vi "PicoScopeospaAWG.vi"(0 "Handle In":i16=16384, 1 "General AWG Settings":T4={"Peak-to-Peak Voltage"=2.0, "Offset Voltage"=0.0, "Wave Type"=17, "Sweep Type"=0, "Cycles"=10, "Trigger Type"=0, "Trigger Source"=4, "sigGenEnabled"=TRUE, "Trigger Enabled"=FALSE, "autoTriggerPicoSeconds"=0} {"Trigger Source" items=["None"=0, "Scope Trigger"=1, "Software Trigger"=4, "Trigger Raw"=5]; "Trigger Type" items=["Rising", "Falling", "Gate High", "Gate Low"]; "Sweep Type" items=["Up", "Down", "Up-Down", "Down-Up"]; "Wave Type" items=["Sine"=17, "Square"=18, "Triangle"=19, "Ramp Up"=20, "Ramp Down"=21, "Sinc"=22, "Gaussian"=23, "Half Sine"=24, "DC"=1024, "PWM"=4096, "White Noise"=8193, "PRBS"=8194, "Arbitrary"=268435456]; "Offset Voltage" format="%#_6p"; "Peak-to-Peak Voltage" format="%#_6p"}, 2 "Standard Waveform Settings":T3={"(Start) Frequency"=1000.0, "Stop Frequency"=5000.0, "Increment"=1.0, "Dwell Time (seconds)"=0.001, "Sweep Enabled"=FALSE} {"Dwell Time (seconds)" format="%#_6p"; "Stop Frequency" min=0.03 max=1000000.0 format="%#_6p"; "(Start) Frequency" min=0.03 max=1000000.0 format="%#_6p"}, 3 "Arbitrary Waveform Settings":T2 {"Index Mode" items=["Single", "Dual", "Quad"]}, 11 "error in":errorcluster, 12 "Duty Cycle":T1={"Use Duty Cycle"=FALSE, "dutyCyclePercent"=20.0}) -> (4 "Handle Out":i16=16384, 13 "Trigger Source Out":u32=4, 14 "Arbitrary\nWaveform Graph":i16[](graph), 15 "error out":errorcluster)   [LabVIEW 2010]
doc: "This VI can be used to control the arbitrary waveform generator. Standard waveforms can be selected or arbitrary waveform can be selected under 'Wave Type'. There are three settings clusters: general settings that apply to both arbitrary and standard waveforms, settings that apply only to standard waveforms and settings that apply only to arbitrary waveforms. It is not necessary to connect all of these clusters if only using arbitrary waveforms or only using standard waveforms are required.\n\nWhen selecting arbitrary waveform, it is necessary to specify a text file containing the wave form. This text file should have a single value on each line in the range -1 to 1. For further information on the settings, see descriptions of ps3000aSetSigGenBuiltIn and ps3000aSetSigGenArbitrary."
uses:
  psospa.dll
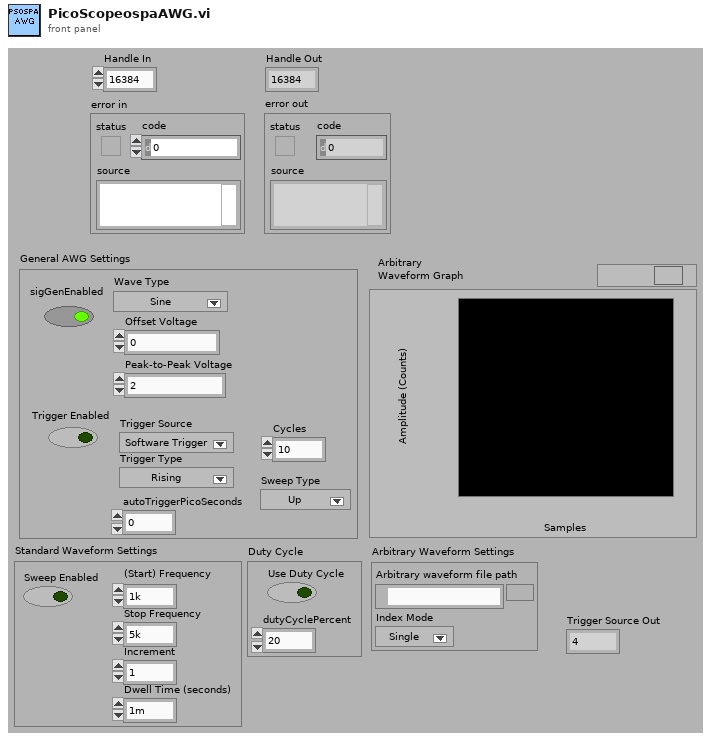
[diagram p1: front panel]
types:
  T1 = cluster{"Use Duty Cycle":bool, "dutyCyclePercent":dbl}
  T2 = cluster{"Arbirary waveform file path":path, "Index Mode":u32}
  T3 = cluster{"(Start) Frequency":dbl, "Stop Frequency":dbl, "Increment":dbl, "Dwell Time (seconds)":dbl, "Sweep Enabled":bool}
  T4 = cluster{"Peak-to-Peak Voltage":dbl, "Offset Voltage":dbl, "Wave Type":u32, "Sweep Type":u32, "Cycles":u64, "Trigger Type":u32, "Trigger Source":u32, "sigGenEnabled":bool, "Trigger Enabled":bool, "autoTriggerPicoSeconds":u64}
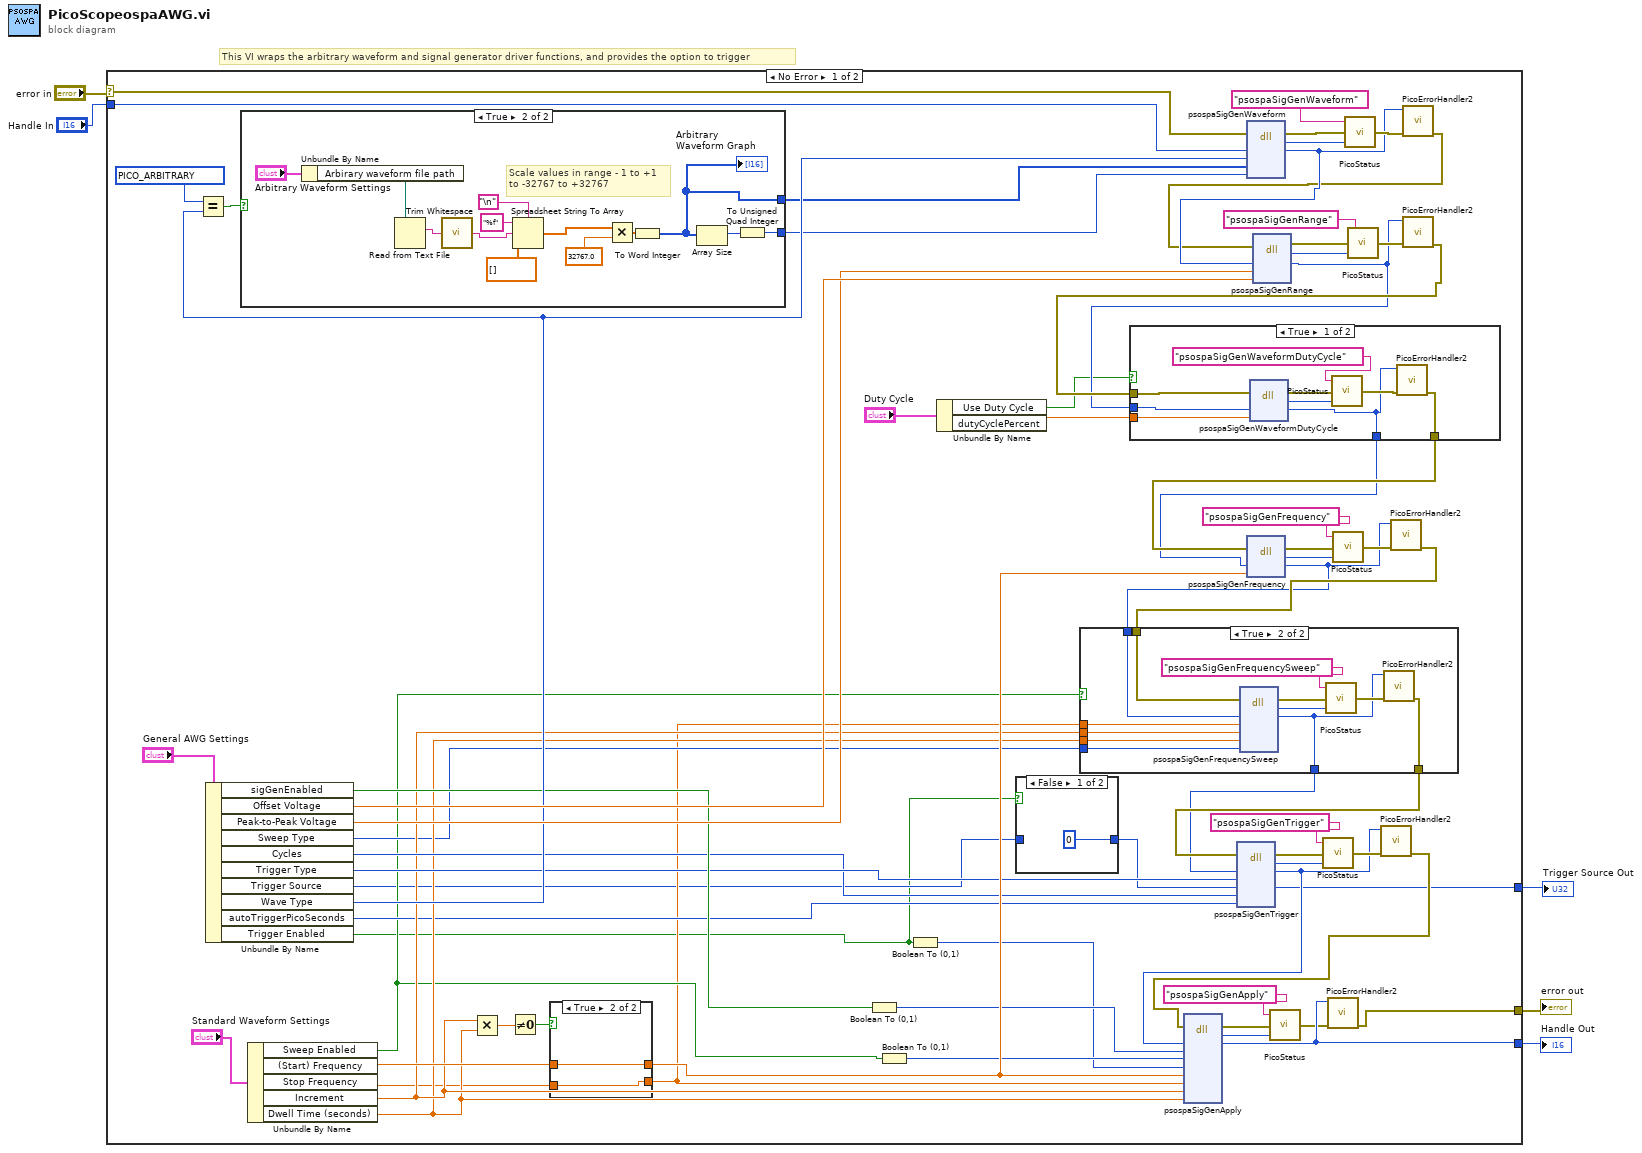
[diagram p0: block diagram]
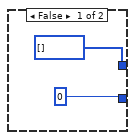
[diagram p4: hidden frame]
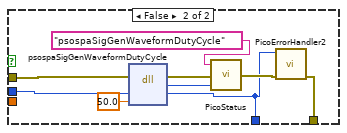
[diagram p5: hidden frame]
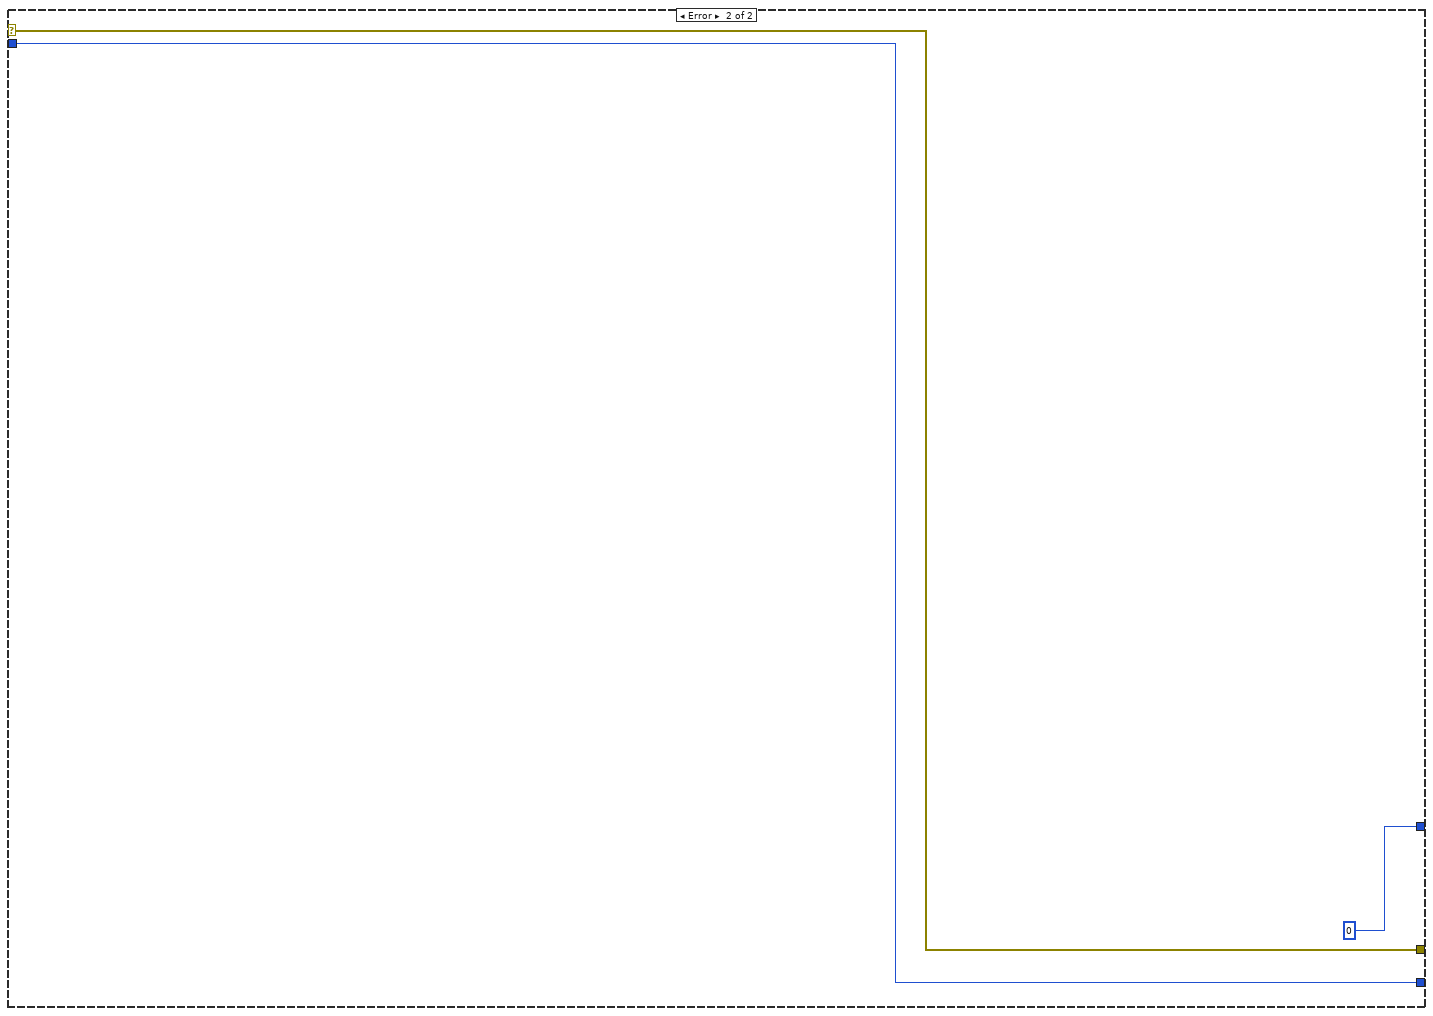
[diagram p7: hidden frame]
diagram:
  # "This VI wraps the arbitrary waveform and signal generator driver functions, and provides the option to trigger"
  n1 = case shown="No Error" "error in" {
    selector: "error in" -> [w69 w129]
    tunnel: [w63 w128] -> w5
    tunnel: "Handle In" -> [w74 w128]
    tunnel: [w62 w129] -> w3
    tunnel: [w9 0] -> w1
    frame No Error {
      w61 = u32 268435456 items=["PICO_ARBITRARY"=268435456]
      n2 = Unbundle By Name("General AWG Settings") -> ("sigGenEnabled"=w32:bool, "Offset Voltage"=w72:dbl, "Peak-to-Peak Voltage"=w71:dbl, "Sweep Type"=w13:u32, "Cycles"=w21:u64, "Trigger Type"=w22:u32, "Trigger Source"=w7:u32, "Wave Type"=w70:u32, "autoTriggerPicoSeconds"=w12:u64, "Trigger Enabled"=w6:bool)
      n3 = Equal?(x=w61, y=w70) -> (x = y?=w33:bool)
      n4 = case shown="True" w33 {
        tunnel: [i16[] [] ("buffer") w94] -> w42
        tunnel: [u64 0 ("bufferLenght") w93] -> w34
        frame False {
        }
        frame True {
          # "Scale values in range - 1 to +1 \nto -32767 to +32767"
          n5 = Unbundle By Name("Arbitrary Waveform Settings") -> ("Arbirary waveform file path"=w99:path)
          n6 = Read from Text File(file (use dialog)=w99) -> (text=w97:string)  [unwired: 3 in, 3 out]
          n7 = call <vilib>:"Trim Whitespace.vi"("string"=w97) -> ("trimmed string"=w96:string)  [unwired: 1 in]
          n8 = Spreadsheet String To Array(delimiter (Tab)="\n", format string="%f", spreadsheet string=w96, array type (2D Dbl)=dbl[] []) -> (array=w101:dbl[])
          n9 = Multiply(x=w101, y=32767.0 ("deltaPhaseIncrement")) -> (x*y=w98:dbl[])
          n10 = To Word Integer(number=w98) -> (16bit integer=w94:i16[])
          "Arbitrary\nWaveform Graph" <- w94
          n11 = Array Size(array=w94) -> (size(s)=w95:i32)
          n12 = To Unsigned Quad Integer(1:w95) -> (0:w93:u64)
        }
      }
      n13 = Unbundle By Name("Standard Waveform Settings") -> ("Sweep Enabled"=w11:bool, "(Start) Frequency"=w67:dbl, "Stop Frequency"=w18:dbl, "Increment"=w20:dbl, "Dwell Time (seconds)"=w19:dbl)
      n14 = Multiply(x=w20, y=w19) -> (x*y=w66:dbl)
      n15 = Not Equal To 0?(x=w66) -> (x != 0?=w65:bool)
      n16 = case shown="True" w65 {
        tunnel: [w124 w126] -> w10
        tunnel: w18 -> [_ w126]
        tunnel: w67 -> [w124 w125]
        tunnel: [w124 w125] -> w64
        frame False {
        }
        frame True {
        }
      }
      n17 = Boolean To (0,1)(Boolean=w32) -> (0, 1=w37:i16)
      n18 = Boolean To (0,1)(Boolean=w11) -> (0, 1=w36:i16)
      n19 = Boolean To (0,1)(Boolean=w6) -> (0, 1=w35:i16)
      n20 = Unbundle By Name("Duty Cycle") -> ("Use Duty Cycle"=w30:bool, "dutyCyclePercent"=w29:dbl)
      n21 = case shown="False" w6 {
        tunnel: [u32 0 ("Trigger Source") w76] -> w8
        tunnel: w7 -> [_ w76]
        frame False {
        }
        frame True {
        }
      }
      n22 = dll-call lib="psospa.dll" fn="psospaSigGenWaveform" ("ps3000.dll:_ps3000_open_unit@0")(error in=w69, "handle"=w74, "waveType"=w70, "buffer"=w42, "bufferLenght"=w34) -> (error out=w58:errorcluster, "PICO_STATUS"=w50:u32, "handle"=w55:i16)  [unwired: 5 in, 1 out]
      n23 = call "PicoStatus.vi"("PICO STATUS"=w50, "error in"=w58, "source"="psospaSigGenWaveform") -> ("error out"=w57:errorcluster)
      n24 = call "PicoErrorHandler2.vi"("error in (no error)"=w57, "handle In"=w55) -> ("error out"=w54:errorcluster)  [unwired: 9 in]
      n25 = dll-call lib="psospa.dll" fn="psospaSigGenRange" ("ps3000.dll:_ps3000_open_unit@0")(error in=w54, "handle"=w55, "peakToPeakVolts"=w71, "offsetVolts"=w72) -> (error out=w53:errorcluster, "PICO_STATUS"=w51:u32, "handle"=w48:i16)  [unwired: 4 in, 1 out]
      n26 = call "PicoStatus.vi"("PICO STATUS"=w51, "error in"=w53, "source"="psospaSigGenRange") -> ("error out"=w52:errorcluster)
      n27 = call "PicoErrorHandler2.vi"("error in (no error)"=w52, "handle In"=w48) -> ("error out"=w49:errorcluster)  [unwired: 9 in]
      n28 = case shown="True" w30 {
        tunnel: w49 -> [w111 w120]
        tunnel: w48 -> [w110 w119]
        tunnel: [w109 w118] -> w46
        tunnel: [w108 w117] -> w45
        tunnel: w29 -> [w106 _]
        frame True {
          n29 = dll-call lib="psospa.dll" fn="psospaSigGenWaveformDutyCycle" ("ps3000.dll:_ps3000_open_unit@0")(error in=w111, "handle"=w110, "dutyCyclePercent"=w106) -> (error out=w114:errorcluster, "PICO_STATUS"=w113:u32, "handle"=w108:i16)  [unwired: 3 in, 1 out]
          n30 = call "PicoStatus.vi"("PICO STATUS"=w113, "error in"=w114, "source"="psospaSigGenWaveformDutyCycle") -> ("error out"=w112:errorcluster)
          n31 = call "PicoErrorHandler2.vi"("error in (no error)"=w112, "handle In"=w108) -> ("error out"=w109:errorcluster)  [unwired: 9 in]
        }
        frame False {
          n32 = dll-call lib="psospa.dll" fn="psospaSigGenWaveformDutyCycle" ("ps3000.dll:_ps3000_open_unit@0")(error in=w120, "handle"=w119, "dutyCyclePercent"=50.0) -> (error out=w123:errorcluster, "PICO_STATUS"=w122:u32, "handle"=w117:i16)  [unwired: 3 in, 1 out]
          n33 = call "PicoStatus.vi"("PICO STATUS"=w122, "error in"=w123, "source"="psospaSigGenWaveformDutyCycle") -> ("error out"=w121:errorcluster)
          n34 = call "PicoErrorHandler2.vi"("error in (no error)"=w121, "handle In"=w117) -> ("error out"=w118:errorcluster)  [unwired: 9 in]
        }
      }
      n35 = dll-call lib="psospa.dll" fn="psospaSigGenFrequency" ("ps3000.dll:_ps3000_open_unit@0")(error in=w46, "handle"=w45, "frequencyHz"=w64) -> (error out=w60:errorcluster, "PICO_STATUS"=w59:u32, "handle"=w16:i16)  [unwired: 3 in, 1 out]
      n36 = call "PicoStatus.vi"("PICO STATUS"=w59, "error in"=w60, "source"="psospaSigGenFrequency") -> ("error out"=w47:errorcluster)
      n37 = call "PicoErrorHandler2.vi"("error in (no error)"=w47, "handle In"=w16) -> ("error out"=w17:errorcluster)  [unwired: 9 in]
      n38 = case shown="True" w11 {
        tunnel: w20 -> [_ w86]
        tunnel: w19 -> [_ w85]
        tunnel: w10 -> [_ w84]
        tunnel: w17 -> [w77 w83]
        tunnel: w16 -> [w78 w82]
        tunnel: [w77 w81] -> w15
        tunnel: [w78 w80] -> w14
        tunnel: w13 -> [_ w79]
        frame False {
        }
        frame True {
          n39 = dll-call lib="psospa.dll" fn="psospaSigGenFrequencySweep" ("ps3000.dll:_ps3000_open_unit@0")(error in=w83, "handle"=w82, "stopFrequencyHz"=w84, "frequencyIncrement"=w86, "dwellTimeSeconds"=w85, "sweepType"=w79) -> (error out=w90:errorcluster, "PICO_STATUS"=w89:u32, "handle"=w80:i16)  [unwired: 6 in, 1 out]
          n40 = call "PicoStatus.vi"("PICO STATUS"=w89, "error in"=w90, "source"="psospaSigGenFrequencySweep") -> ("error out"=w88:errorcluster)
          n41 = call "PicoErrorHandler2.vi"("error in (no error)"=w88, "handle In"=w80) -> ("error out"=w81:errorcluster)  [unwired: 9 in]
        }
      }
      n42 = dll-call lib="psospa.dll" fn="psospaSigGenTrigger" ("ps3000.dll:_ps3000_open_unit@0")(error in=w15, "handle"=w14, "triggerType"=w22, "triggerSource"=w8, "cycles"=w21, "autoTriggerPicoSeconds"=w12) -> (error out=w28:errorcluster, "PICO_STATUS"=w27:u32, "handle"=w23:i16, "triggerSource"=w9:u32)  [unwired: 5 in, 1 out]
      n43 = call "PicoStatus.vi"("PICO STATUS"=w27, "error in"=w28, "source"="psospaSigGenTrigger") -> ("error out"=w26:errorcluster)
      n44 = call "PicoErrorHandler2.vi"("error in (no error)"=w26, "handle In"=w23) -> ("error out"=w24:errorcluster)  [unwired: 9 in]
      n45 = dll-call lib="psospa.dll" fn="psospaSigGenApply" ("ps3000.dll:_ps3000_open_unit@0")(error in=w24, "handle"=w23, "sigGenEnabled"=w37, "sweepEnabled"=w36, "triggerEnabled"=w35, "frequency"=w64, "stopFrequency"=w10, "frequencyIncrement"=w20, "dwellTime"=w19) -> (error out=w41:errorcluster, "PICO_STATUS"=w40:u32, "handle"=w63:i16)  [unwired: 9 in, 1 out]
      n46 = call "PicoStatus.vi"("PICO STATUS"=w40, "error in"=w41, "source"="psospaSigGenApply") -> ("error out"=w39:errorcluster)
      n47 = call "PicoErrorHandler2.vi"("error in (no error)"=w39, "handle In"=w63) -> ("error out"=w62:errorcluster)  [unwired: 9 in]
    }
    frame Error {
    }
  }
  "Handle Out" <- w5
  "error out" <- w3
  "Trigger Source Out" <- w1
